vi "Petrol filling.vi"() -> ()   [LabVIEW 2024]
panel:
  in  "Low pass value":dbl
  out "Petrol in litres":dbl
  in  "Enter Amount":dbl
  # "Overview: Demonstrates how the Numeric functions used.\nInstructions:\n1. Enter the amount.\n2.Run the VI"
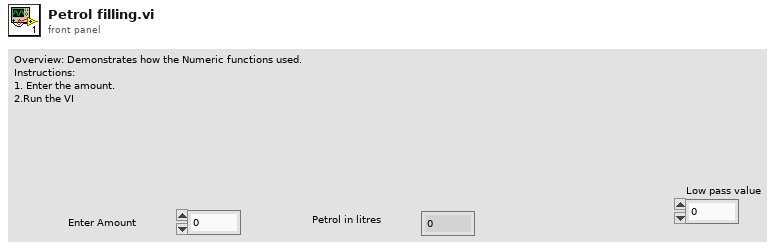
[diagram p1: front panel]
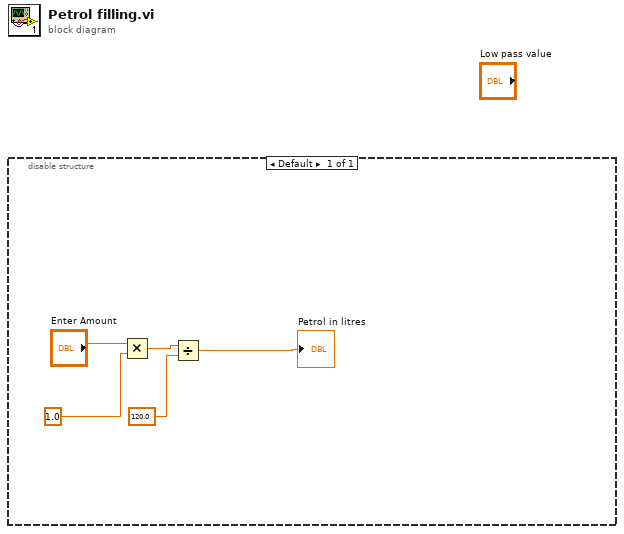
[diagram p0: block diagram]
diagram:
  n1 = disable-structure shown="Default" {
    frame Enabled {
      n2 = Multiply(x="Enter Amount", y=1.0 ("Enter Amount")) -> (x*y=w3:dbl)
      n3 = Divide(x=w3, y=120.0) -> (x/y=→"Petrol in litres":dbl)
    }
  }
